vi "CONTROL.vi"(0 "Boolean in":refnum<vi>, 1 "reference":refnum<vi>, 2 "reference 2":refnum<vi>, 3 "reference 3":refnum<vi>, 4 "reference 4":refnum<vi>, 5 "reference 5":refnum<vi>, 6 "reference 8":refnum<vi>, 7 "reference 6":refnum<vi>, 8 "X Axis":i32, 9 "reference 7":refnum<vi>, 10 "Y Axis":i32) -> (11 "Foward":bool, 12 "Right":bool, 13 "FR":bool, 14 "Reverse":bool, 15 "FL":bool, 16 "RR":bool, 17 "RL":bool, 18 "stay":bool, 19 "Left":bool)   [LabVIEW 2019]
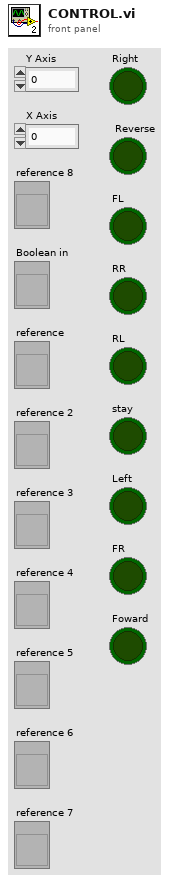
[diagram p1: front panel]
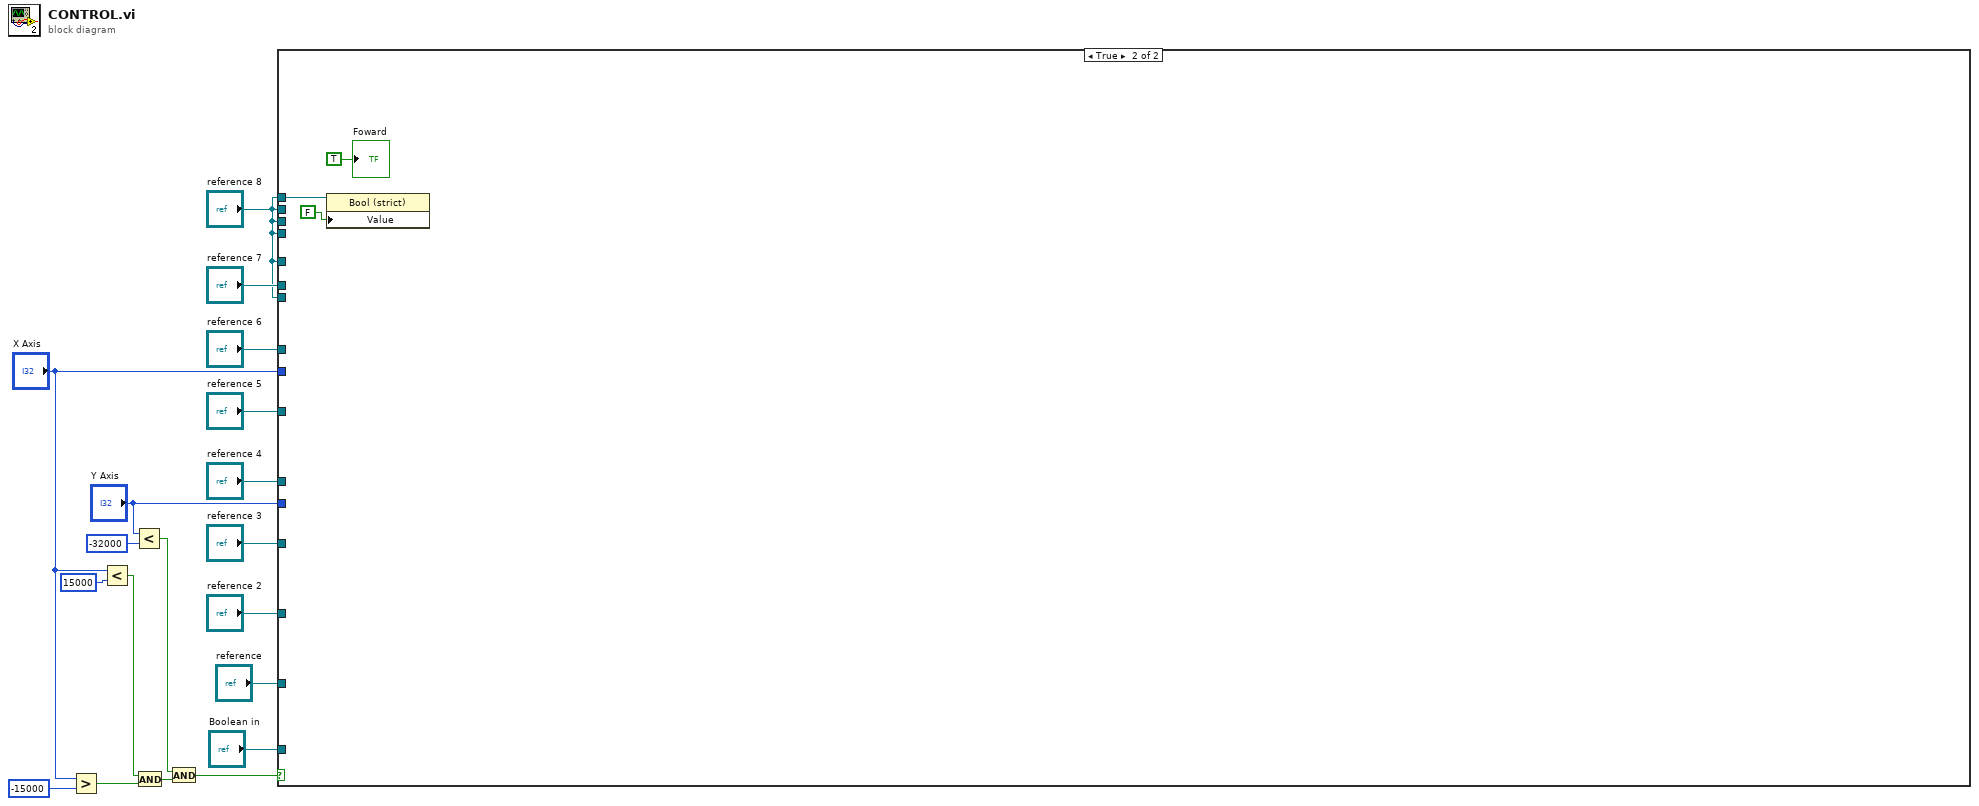
[diagram p0: block diagram]
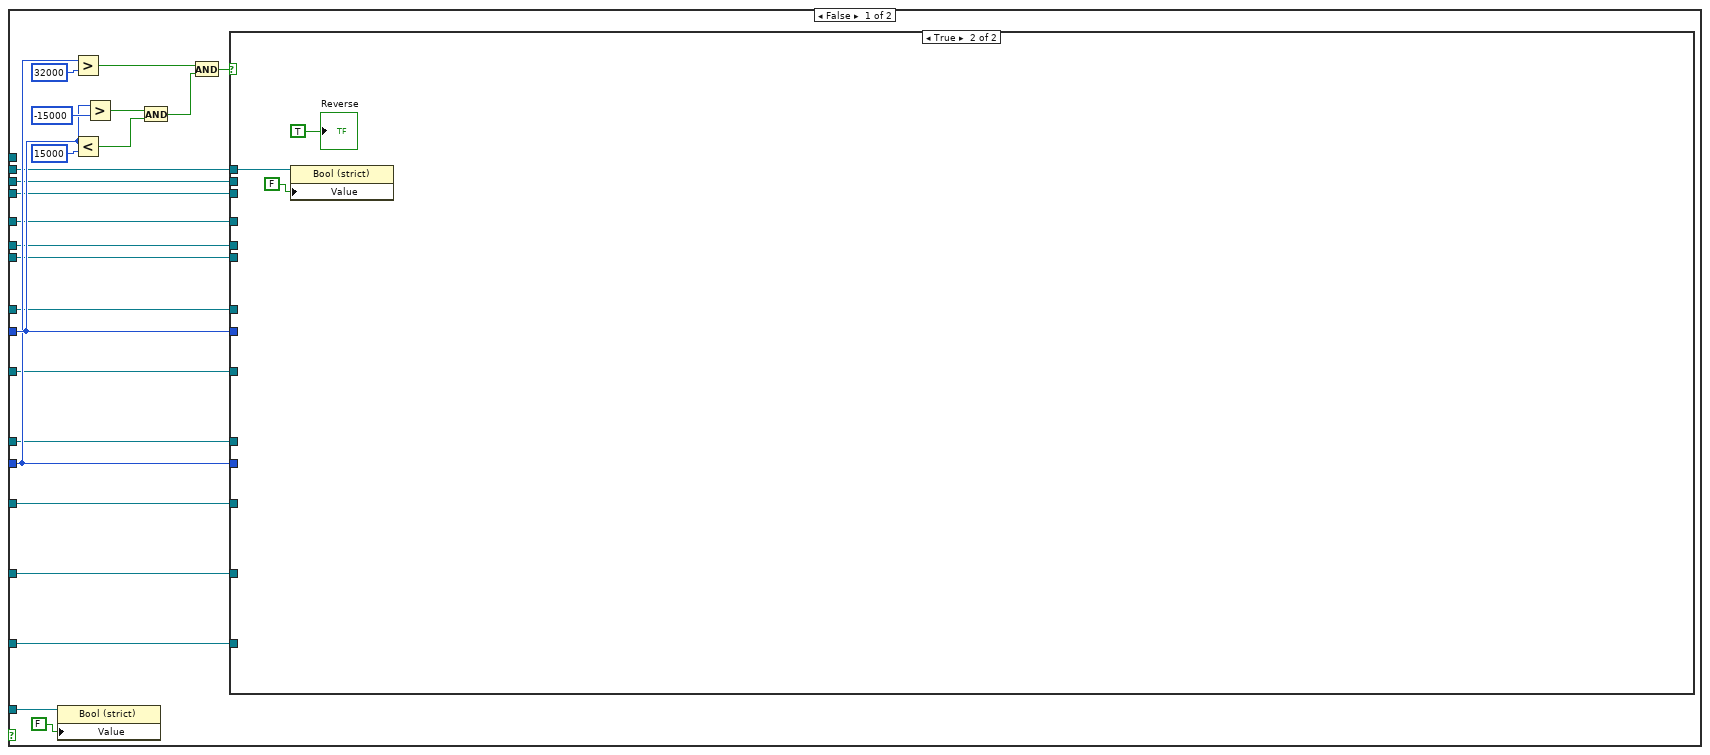
[diagram p2: hidden frame]
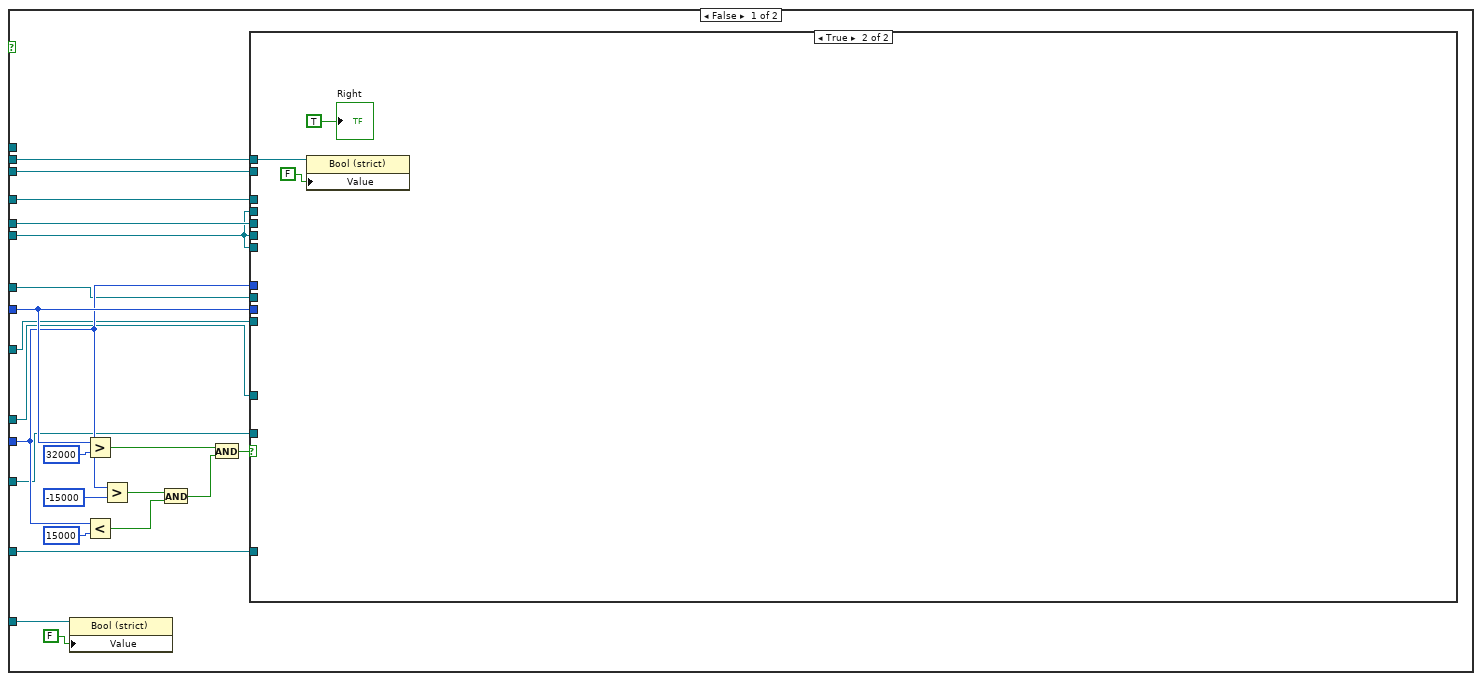
[diagram p3: hidden frame]
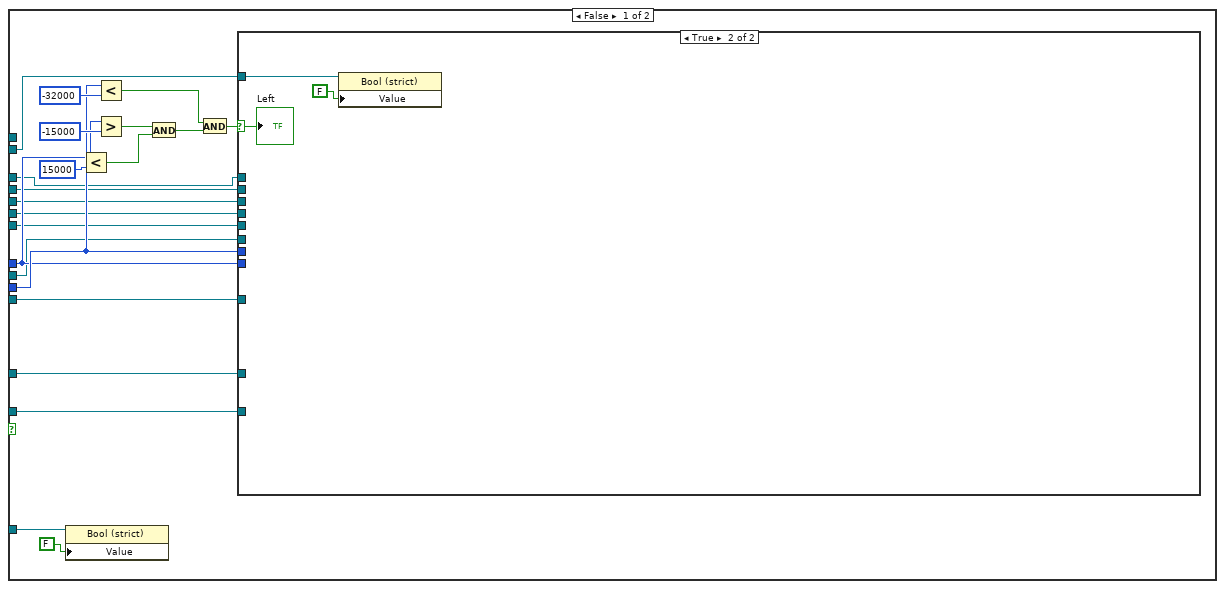
[diagram p4: hidden frame]
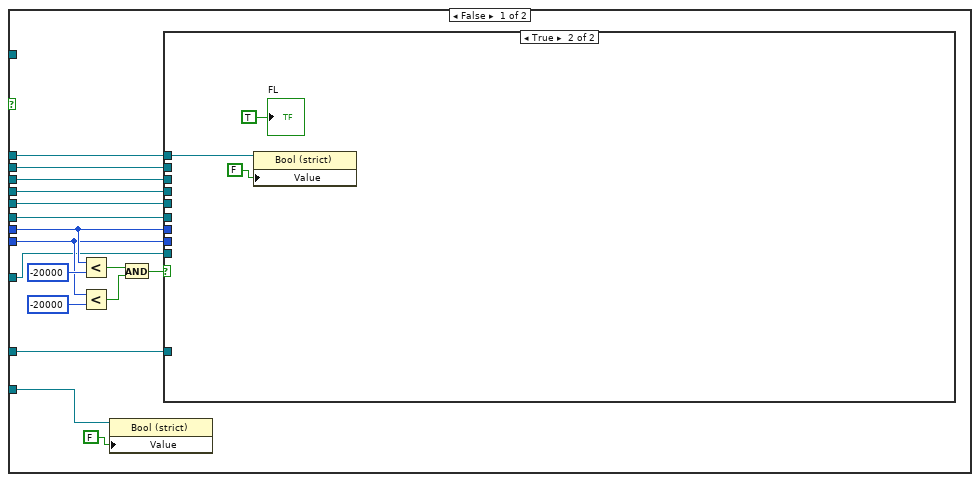
[diagram p5: hidden frame]
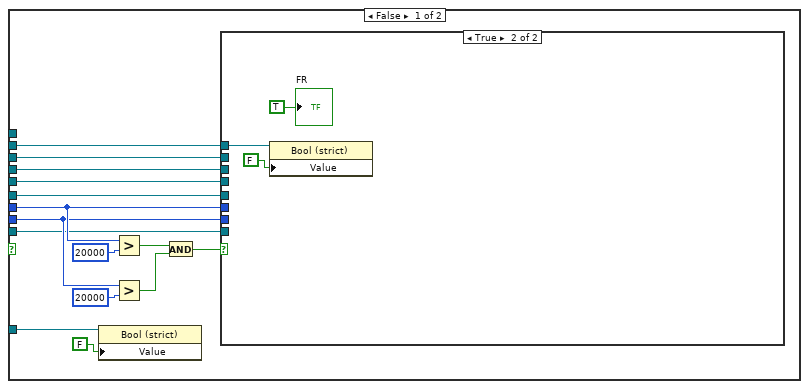
[diagram p6: hidden frame]
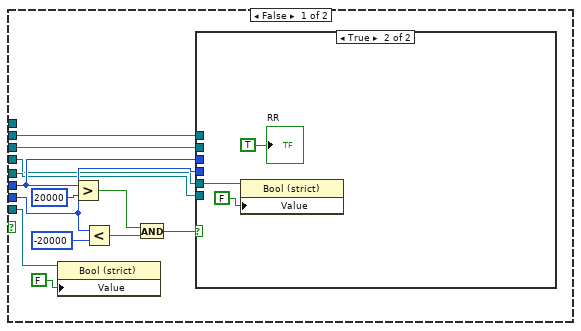
[diagram p7: hidden frame]
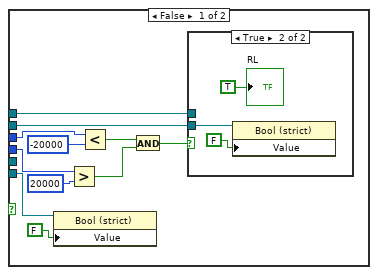
[diagram p8: hidden frame]
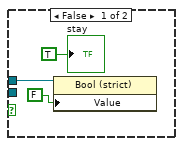
[diagram p9: hidden frame]
diagram:
  n1 = Greater?(x="X Axis", y=-15000) -> (0:w18:bool)
  n2 = Less?(x="X Axis", y=15000) -> (x < y?=w17:bool)
  n3 = Less?(x="Y Axis", y=-32000) -> (x < y?=w13:bool)
  n4 = And(x=w17, y=w18) -> (x .and. y?=w19:bool)
  n5 = And(x=w13, y=w19) -> (x .and. y?=w14:bool)
  n6 = case shown="True" w14 {
    tunnel: "Y Axis" -> [w33 _]
    tunnel: "X Axis" -> [w40 _]
    tunnel: "reference" -> [w32 _]
    tunnel: "reference 2" -> [w31 _]
    tunnel: "reference 3" -> [w30 _]
    tunnel: "reference 4" -> [w29 _]
    tunnel: "reference 5" -> [w28 _]
    tunnel: "reference 6" -> [w27 _]
    tunnel: "reference 7" -> [w26 _]
    tunnel: "reference 8" -> [w25 _]
    tunnel: "reference 8" -> [w24 _]
    tunnel: "reference 8" -> [w23 _]
    tunnel: "reference 8" -> [w22 _]
    tunnel: "reference 8" -> [w21 _]
    tunnel: "Boolean in" -> [w20 _]
    tunnel: "reference 8" -> [_ w168]
    frame False {
      n7 = property class="Bool (strict)"(reference=w20, "Value"=FALSE ("Front")) -> ()  [unwired: 1 in, 2 out]
      n8 = Greater?(x=w33, y=32000) -> (0:w35:bool)
      n9 = Less?(x=w40, y=15000) -> (x < y?=w37:bool)
      n10 = Greater?(x=w40, y=-15000) -> (0:w38:bool)
      n11 = And(x=w38, y=w37) -> (x .and. y?=w36:bool)
      n12 = And(x=w35, y=w36) -> (x .and. y?=w34:bool)
      n13 = case shown="True" w34 {
        tunnel: w40 -> [w63 _]
        tunnel: w33 -> [w55 _]
        tunnel: w32 -> [w54 _]
        tunnel: w31 -> [w53 _]
        tunnel: w30 -> [w52 _]
        tunnel: w29 -> [w51 _]
        tunnel: w28 -> [w50 _]
        tunnel: w27 -> [w49 _]
        tunnel: w26 -> [w48 _]
        tunnel: w25 -> [w47 _]
        tunnel: w24 -> [w46 _]
        tunnel: w23 -> [w45 _]
        tunnel: w22 -> [w44 _]
        tunnel: w21 -> [_ w165]
        frame False {
          n14 = property class="Bool (strict)"(reference=w54, "Value"=FALSE ("Reverse")) -> ()  [unwired: 1 in, 2 out]
          n15 = Greater?(x=w63, y=32000) -> (0:w57:bool)
          n16 = Less?(x=w55, y=15000) -> (x < y?=w59:bool)
          n17 = Greater?(x=w55, y=-15000) -> (0:w60:bool)
          n18 = And(x=w60, y=w59) -> (x .and. y?=w58:bool)
          n19 = And(x=w57, y=w58) -> (x .and. y?=w56:bool)
          n20 = case shown="True" w56 {
            tunnel: w63 -> [w78 _]
            tunnel: w55 -> [w77 _]
            tunnel: w53 -> [w76 _]
            tunnel: w52 -> [w75 _]
            tunnel: w51 -> [w74 _]
            tunnel: w50 -> [w73 _]
            tunnel: w49 -> [w72 _]
            tunnel: w48 -> [w71 _]
            tunnel: w47 -> [w70 _]
            tunnel: w47 -> [w69 _]
            tunnel: w47 -> [w68 _]
            tunnel: w46 -> [w67 _]
            tunnel: w45 -> [w66 _]
            tunnel: w44 -> [_ w162]
            frame False {
              n21 = property class="Bool (strict)"(reference=w76, "Value"=FALSE ("Right")) -> ()  [unwired: 1 in, 2 out]
              n22 = Less?(x=w77, y=15000) -> (x < y?=w82:bool)
              n23 = Less?(x=w78, y=-32000) -> (x < y?=w80:bool)
              n24 = Greater?(x=w77, y=-15000) -> (0:w83:bool)
              n25 = And(x=w83, y=w82) -> (x .and. y?=w79:bool)
              n26 = And(x=w80, y=w79) -> (x .and. y?=w81:bool)
              n27 = case shown="True" w81 {
                selector: w81 -> [_ w161]
                tunnel: w78 -> [w98 _]
                tunnel: w77 -> [w97 _]
                tunnel: w75 -> [w96 _]
                tunnel: w74 -> [w95 _]
                tunnel: w73 -> [w94 _]
                tunnel: w72 -> [w93 _]
                tunnel: w71 -> [w92 _]
                tunnel: w70 -> [w91 _]
                tunnel: w69 -> [w90 _]
                tunnel: w68 -> [w89 _]
                tunnel: w67 -> [w88 _]
                tunnel: w66 -> [_ w159]
                frame False {
                  n28 = Less?(x=w98, y=-20000) -> (x < y?=w100:bool)
                  n29 = Less?(x=w97, y=-20000) -> (x < y?=w101:bool)
                  n30 = property class="Bool (strict)"(reference=w96, "Value"=FALSE ("Left")) -> ()  [unwired: 1 in, 2 out]
                  n31 = And(x=w100, y=w101) -> (x .and. y?=w99:bool)
                  n32 = case shown="True" w99 {
                    tunnel: w98 -> [w113 _]
                    tunnel: w97 -> [w112 _]
                    tunnel: w95 -> [w111 _]
                    tunnel: w94 -> [w110 _]
                    tunnel: w93 -> [w109 _]
                    tunnel: w92 -> [w108 _]
                    tunnel: w91 -> [w107 _]
                    tunnel: w90 -> [w106 _]
                    tunnel: w89 -> [w105 _]
                    tunnel: w88 -> [_ w156]
                    frame False {
                      n33 = property class="Bool (strict)"(reference=w111, "Value"=FALSE ("FL")) -> ()  [unwired: 1 in, 2 out]
                      n34 = Greater?(x=w113, y=20000) -> (0:w116:bool)
                      n35 = Greater?(x=w112, y=20000) -> (0:w117:bool)
                      n36 = And(x=w116, y=w117) -> (x .and. y?=w115:bool)
                      n37 = case shown="True" w115 {
                        tunnel: w113 -> [w126 _]
                        tunnel: w112 -> [w125 _]
                        tunnel: w110 -> [w124 _]
                        tunnel: w109 -> [w123 _]
                        tunnel: w108 -> [w122 _]
                        tunnel: w107 -> [w121 _]
                        tunnel: w106 -> [w120 _]
                        tunnel: w105 -> [_ w153]
                        frame False {
                          n38 = property class="Bool (strict)"(reference=w124, "Value"=FALSE ("FR")) -> ()  [unwired: 1 in, 2 out]
                          n39 = Greater?(x=w126, y=20000) -> (0:w129:bool)
                          n40 = Less?(x=w125, y=-20000) -> (x < y?=w130:bool)
                          n41 = And(x=w129, y=w130) -> (x .and. y?=w127:bool)
                          n42 = case shown="True" w127 {
                            tunnel: w126 -> [w138 _]
                            tunnel: w125 -> [w137 _]
                            tunnel: w123 -> [w135 _]
                            tunnel: w122 -> [w134 _]
                            tunnel: w121 -> [w133 _]
                            tunnel: w120 -> [_ w150]
                            frame False {
                              n43 = property class="Bool (strict)"(reference=w135, "Value"=FALSE ("RR")) -> ()  [unwired: 1 in, 2 out]
                              n44 = Greater?(x=w137, y=20000) -> (0:w141:bool)
                              n45 = Less?(x=w138, y=-20000) -> (x < y?=w140:bool)
                              n46 = And(x=w140, y=w141) -> (x .and. y?=w136:bool)
                              n47 = case shown="True" w136 {
                                tunnel: w134 -> [w144 _]
                                tunnel: w133 -> [_ w147]
                                frame False {
                                n48 = property class="Bool (strict)"(reference=w144, "Value"=FALSE ("RL")) -> ()  [unwired: 1 in, 2 out]
                                "stay" <- TRUE ("Left 2")
                                }
                                frame True {
                                n49 = property class="Bool (strict)"(reference=w147, "Value"=FALSE ("stay")) -> ()  [unwired: 1 in, 2 out]
                                "RL" <- TRUE ("RL")
                                }
                              }
                            }
                            frame True {
                              n50 = property class="Bool (strict)"(reference=w150, "Value"=FALSE ("stay")) -> ()  [unwired: 1 in, 2 out]
                              "RR" <- TRUE ("RR")
                            }
                          }
                        }
                        frame True {
                          n51 = property class="Bool (strict)"(reference=w153, "Value"=FALSE ("stay")) -> ()  [unwired: 1 in, 2 out]
                          "FR" <- TRUE ("FR")
                        }
                      }
                    }
                    frame True {
                      n52 = property class="Bool (strict)"(reference=w156, "Value"=FALSE ("stay")) -> ()  [unwired: 1 in, 2 out]
                      "FL" <- TRUE ("FL")
                    }
                  }
                }
                frame True {
                  n53 = property class="Bool (strict)"(reference=w159, "Value"=FALSE ("stay")) -> ()  [unwired: 1 in, 2 out]
                  "Left" <- w161
                }
              }
            }
            frame True {
              n54 = property class="Bool (strict)"(reference=w162, "Value"=FALSE ("stay")) -> ()  [unwired: 1 in, 2 out]
              "Right" <- TRUE ("Right")
            }
          }
        }
        frame True {
          n55 = property class="Bool (strict)"(reference=w165, "Value"=FALSE ("stay")) -> ()  [unwired: 1 in, 2 out]
          "Reverse" <- TRUE ("Reverse")
        }
      }
    }
    frame True {
      n56 = property class="Bool (strict)"(reference=w168, "Value"=FALSE ("stay")) -> ()  [unwired: 1 in, 2 out]
      "Foward" <- TRUE ("Front")
    }
  }
